vi "command.vi"(8 "error in (no error)":errorcluster, 10 "command":string, 11 "NEXUS in":refnum<class "NEXUS.lvclass">) -> (0 "error out":errorcluster, 2 "response":string, 3 "NEXUS out":refnum<class "NEXUS.lvclass">)   [LabVIEW 2019, in "NEXUS.lvclass"]
uses:
  NEXUS.lvclass
  Instrumento/Instrumento.lvclass
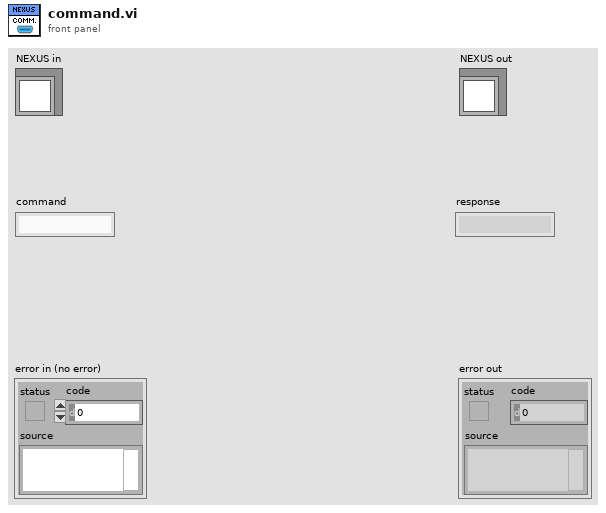
[diagram p1: front panel]
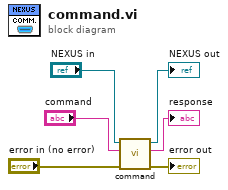
[diagram p0: block diagram]
diagram:
  n1 = call-parent "command.vi"("error in (no error)"="error in (no error)", "command"="command", "Instrumento in"="NEXUS in") -> ("error out"=→"error out":errorcluster, "response"=→"response":string, "Instrumento out"=→"NEXUS out":refnum<class "NEXUS.lvclass">)  [unwired: 6 in]
